vi "Prueba 2 Version 3.vi"() -> ()   [LabVIEW 2013]
panel:
  out "Contador":dbl
  out "Temperatura Mayor":dbl
  out "Temperatura Promedio":dbl
  out "Mucha Calor":bool
  out "Thermometer":i32(slide) scale=0.0..60.0
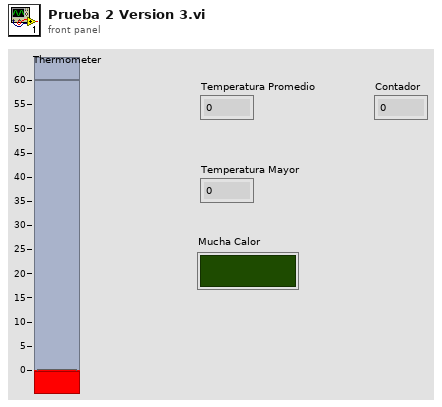
[diagram p1: front panel]
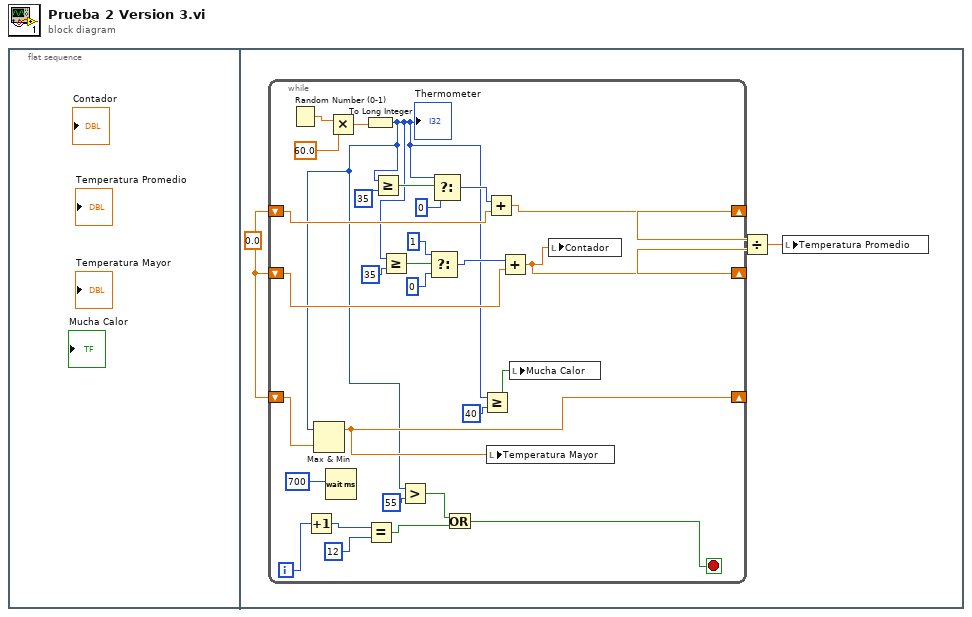
[diagram p0: block diagram]
diagram:
  n1 = flat-sequence {
    frame #0 {
    }
    frame #1 {
      w1 = 0.0
      n2 = while {
        shift-right: [w25] -> w3
        shift-left: w1 -> [w26]
        shift-right: [w18] -> w4
        shift-left: w1 -> [w19]
        shift-right: [w14] -> _
        shift-left: w1 -> [w15]
        i -> [w10]
        stop <- w6 stop-if-true
        n3 = Random Number (0-1)() -> (number: 0 to 1=w33:dbl)
        n4 = Increment(x=w10) -> (x+1=w12:i32)
        n5 = Wait (ms)(milliseconds to wait=700) -> ()  [unwired: 1 out]
        n6 = Multiply(x=w33, y=60.0) -> (x*y=w31:dbl)
        n7 = To Long Integer(number=w31) -> (32bit integer=w5:i32)
        "Thermometer" <- w5
        n8 = Max & Min(x=w5, y=w15) -> (max(x,y)=w14:dbl)  [unwired: 1 out]
        n9 = Equal?(x=w12, y=12) -> (x = y?=w8:bool)
        n10 = Greater Or Equal?(x=w5, y=35) -> (x >= y?=w29:bool)
        n11 = Greater Or Equal?(x=w5, y=35) -> (x >= y?=w23:bool)
        n12 = Greater?(x=w5, y=55) -> (0:w7:bool)
        n13 = Select(t=1, s=w23, f=0) -> (s? t:f=w20:i32)
        n14 = Select(t=w5, s=w29, f=0) -> (s? t:f=w27:i32)
        n15 = Or(x=w7, y=w8) -> (x .or. y?=w6:bool)
        n16 = Greater Or Equal?(x=w5, y=40) -> (x >= y?=w16:bool)
        n17 = Add(x=w27, y=w26) -> (x+y=w25:dbl)
        n18 = local write "Temperatura Mayor"(w14) -> ()
        n19 = Add(x=w20, y=w19) -> (x+y=w18:dbl)
        n20 = local write "Mucha Calor"(w16) -> ()
        n21 = local write "Contador"(w18) -> ()
      }
      n22 = Divide(x=w3, y=w4) -> (x/y=w2:dbl)
      n23 = local write "Temperatura Promedio"(w2) -> ()
    }
  }
